vi "Roll Row.vi"(10 "Reverse":bool, 11 "Row In":T1[](array[typedef])) -> (3 "Row Out":T1[](array[typedef]))   [LabVIEW 2023]
uses:
  ENUM_Type.ctl
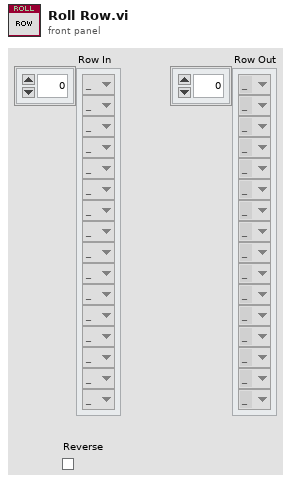
[diagram p1: front panel]
types:
  T1 = typedef "ENUM_Type.ctl" = enum16{"_", "O", "#"}
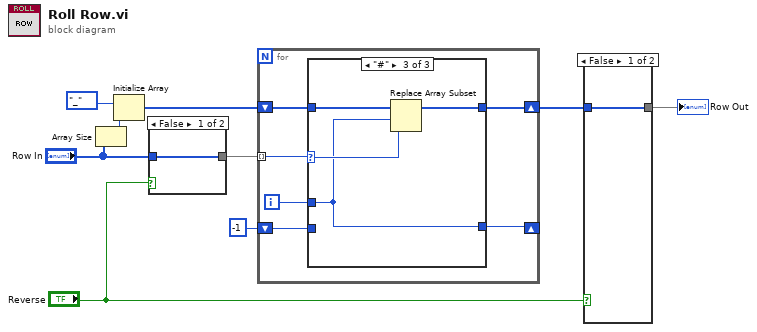
[diagram p0: block diagram]
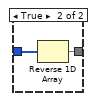
[diagram p2: hidden frame]
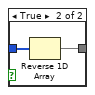
[diagram p3: hidden frame]
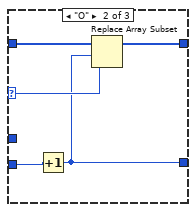
[diagram p5: hidden frame]
diagram:
  n1 = Array Size(array="Row In") -> (size(s)=w5:i32)
  n2 = Initialize Array(ENUM_Type."_" ("Enum"), w5) -> (w6:T1[])
  n3 = case shown="False" "Reverse" {
    tunnel: "Row In" -> [w10 w12]
    tunnel: [w10 w11] -> w3
    frame False {
    }
    frame True {
      n4 = Reverse 1D Array(array=w12) -> (reversed array=w11:T1[])
    }
  }
  n5 = for {
    shift-right: [w14] -> w9
    shift-left: w6 -> [w16]
    shift-right: [w15] -> _
    shift-left: -1 -> [w17]
    tunnel: w3 -> [w18] mode=indexing
    i -> [w13]
    n6 = case shown="\"#\"" w18 {
      selector: w18 -> [_ w22 w27]
      tunnel: w17 -> [w19 w25 _]
      tunnel: w16 -> [w20 w24 w29]
      tunnel: [w19 w21 w26] -> w15
      tunnel: [w20 w23 w28] -> w14
      tunnel: w13 -> [_ _ w26]
      frame "_" {
      }
      frame "O" {
        n7 = Increment(x=w25) -> (x+1=w21:i32)
        n8 = Replace Array Subset(array=w24, new element=w22, index=w21) -> (w23:T1[])
      }
      frame "#" {
        n9 = Replace Array Subset(array=w29, new element=w27, index=w26) -> (w28:T1[])
      }
    }
  }
  n10 = case shown="False" "Reverse" {
    tunnel: w9 -> [w30 w32]
    tunnel: [w30 w31] -> w2
    frame False {
    }
    frame True {
      n11 = Reverse 1D Array(array=w32) -> (reversed array=w31:T1[])
    }
  }
  "Row Out" <- w2
